vi "Set Sender.vi"(10 "Sender":refnum<class "Sender.lvclass">, 11 "Teardown Error Msg in":refnum<class "Teardown Error Msg.lvclass">) -> (3 "Teardown Error Msg out":refnum<class "Teardown Error Msg.lvclass">)   [LabVIEW 2020, in "jettl.lvlib" / "Teardown Error Msg.lvlib" / "Teardown Error Msg.lvclass"]
uses:
  Teardown Error Msg.lvclass
  Sender/Sender/Sender.lvclass
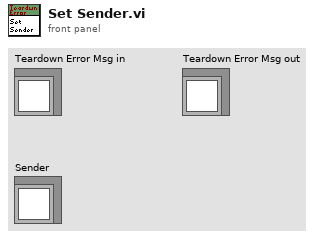
[diagram p1: front panel]
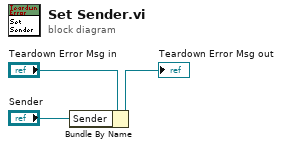
[diagram p0: block diagram]
diagram:
  n1 = Bundle By Name(cluster="Teardown Error Msg in", "Sender"="Sender") -> (→"Teardown Error Msg out":refnum<class "Teardown Error Msg.lvclass">)
